vi "PIO.Set Window Base Address.vi"(8 "error in (no error)":errorcluster, 10 "Local Base Address":u32 format="%.0x", 11 "GE 5565PIORC in":refnum<class "GE 5565PIORC Old.lvclass">) -> (0 "error out":errorcluster, 3 "GE 5565PIORC out":refnum<class "GE 5565PIORC Old.lvclass">)   [LabVIEW 2016, in "GE 5565PIORC Old.lvclass"]
uses:
  GE 5565PIORC Old.lvclass
  GE 5565PIORC Old.lvclass/GE 5565PIORC Old.ctl
  Registers/Local Configuration.Get Register Offset.vi
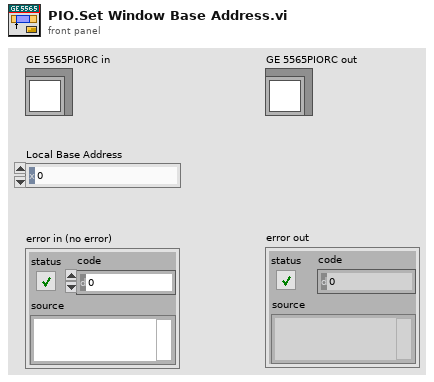
[diagram p1: front panel]
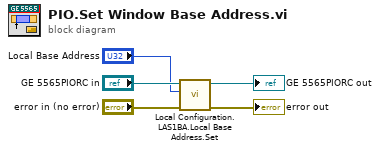
[diagram p0: block diagram]
diagram:
  n1 = call "Local Configuration.LAS1BA.Local Base Address.Set.vi"("error in (no error)"="error in (no error)", "Local Base Address"="Local Base Address", "GE 5565PIORC"="GE 5565PIORC in") -> ("error out"=→"error out":errorcluster, "GE 5565PIORC out"=→"GE 5565PIORC out":refnum<class "GE 5565PIORC Old.lvclass">)  [unwired: 7 in]
